vi "WriteFile.vi"(6 "Refresh Time":dbl, 8 "Error In":errorcluster, 9 "Measurements":T1 {"Measurement Type (0: Voltage RMS L-N)" items=["Voltage RMS L-N", "Voltage RMS L-L", "Frequency", "Current RMS", "Current Peak", "Crest Factor", "Power Factor", "Power VA", "Real Power", "Voltage Harmonic THD", "Voltage Harmonic OHD", "Voltage Harmonic EHD", "Current Harmonic THD", "Current Harmonic OHD", "Current Harmonic EHD"]; "Channel Name(1: A)" items=["A"=1, "B"=2, "C"=3]}, 10 "Load Settings":T2 {"Arbitrary Waveform"."Waveform Number (2: Arbitrary Waveform2)" items=["Arbitrary Waveform 2"=2, "Arbitrary Waveform 3"=3, "Arbitrary Waveform 4"=4, "Arbitrary Waveform 5"=5, "Arbitrary Waveform 6"=6, "Arbitrary Waveform 7"=7, "Arbitrary Waveform 8"=8, "Arbitrary Waveform 9"=9, "Arbitrary Waveform 10"=10, "Arbitrary Waveform 11"=11, "Arbitrary Waveform 12"=12, "Arbitrary Waveform 13"=13, "Arbitrary Waveform 14"=14, "Arbitrary Waveform 15"=15, "Arbitrary Waveform 16"=16, "Arbitrary Waveform 17"=17, "Arbitrary Waveform 18"=18, "Arbitrary Waveform 19"=19, "Arbitrary Waveform 20"=20, "Arbitrary Waveform 21"=21, "Arbitrary Waveform 22"=22]; "Waveform"."Waveform (1: Sine)" items=["Sine"=1, "Arbitrary Waveform 2"=2, "Arbitrary Waveform 3"=3, "Arbitrary Waveform 4"=4, "Arbitrary Waveform 5"=5, "Arbitrary Waveform 6"=6, "Arbitrary Waveform 7"=7, "Arbitrary Waveform 8"=8, "Arbitrary Waveform 9"=9, "Arbitrary Waveform 10"=10, "Arbitrary Waveform 11"=11, "Arbitrary Waveform 12"=12, "Arbitrary Waveform 13"=13, "Arbitrary Waveform 14"=14, "Arbitrary Waveform 15"=15, "Arbitrary Waveform 16"=16, "Arbitrary Waveform 17"=17, "Arbitrary Waveform 18"=18, "Arbitrary Waveform 19"=19, "Arbitrary Waveform 20"=20, "Arbitrary Waveform 21"=21, "Arbitrary Waveform 22"=22]; "Waveform"."Channel Name (1: A)" items=["A"=1, "B"=2, "C"=3]; "Frequency"."Frequency Range (600Hz)" items=["150 Hz", "300 Hz", "600 Hz", "1200 Hz"]; "Range Control (0: Auto)" items=["Auto", "<110 V", "110 V -120.9 V", "121 V - 130.9 V", "> 131 V"]; "Configure Output"."Form (3: Three)" items=["Single", "Split", "Three"]; "Configure Output"."Coupling  (0: Direct)" items=["Direct", "Transformer"]}, 11 "refnum":T3) -> (0 "error out":errorcluster)   [LabVIEW 2018, in "AcPwrPlugins.lvlib" / "PacificPowerSource.lvclass"]
doc: "This VI writes the properties to the INI configuration file."
uses:
  PacificPowerSource.lvclass
  <vilib>/Utility/config.llb/Config Data RefNum.ctl
  TypeDefs/DeviceSettings.ctl
  TypeDefs/Measurements.ctl
  <vilib>/Utility/config.llb/NI_LVConfig.lvlib
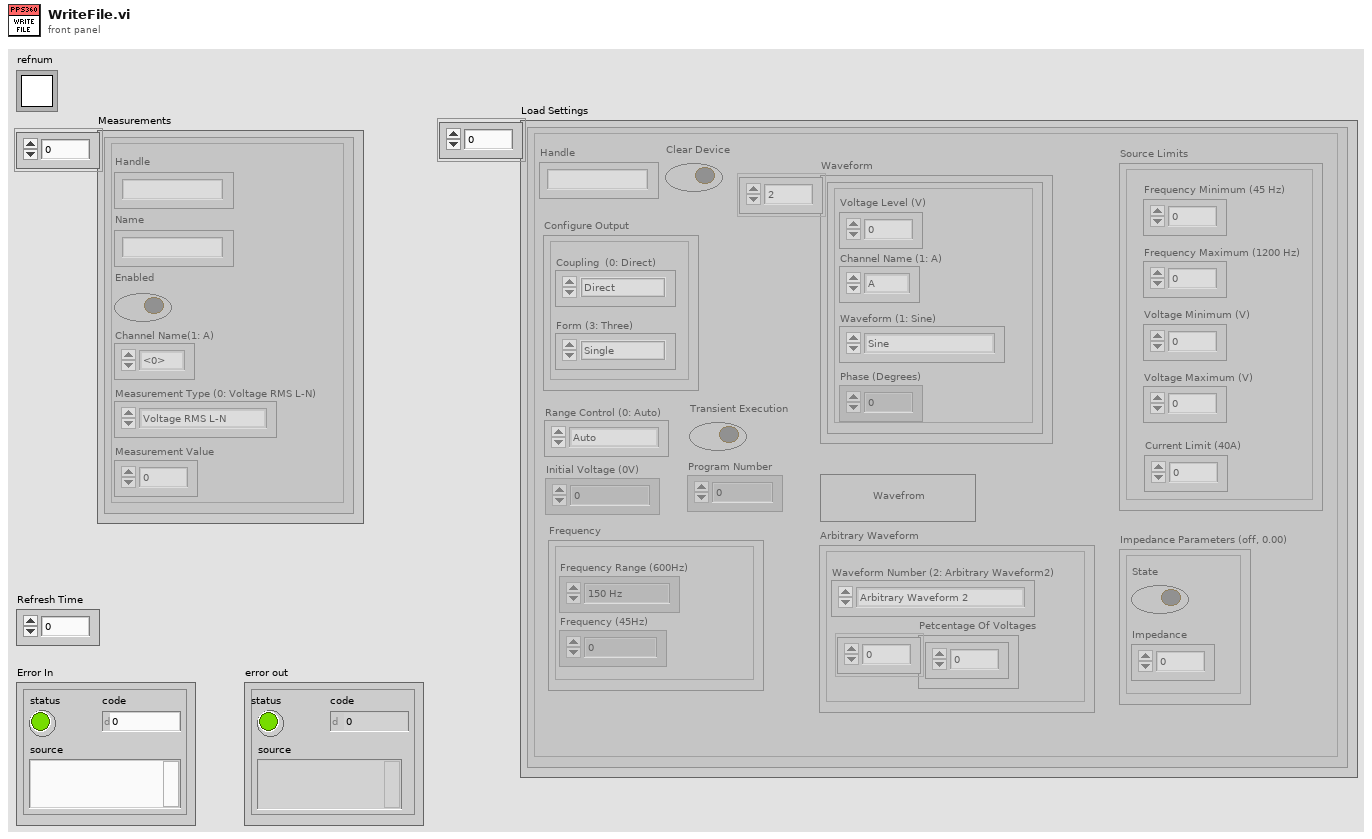
[diagram p1: front panel]
types:
  T1 = typedef "AcPwrPlugins.lvlib/PacificPowerSource.lvclass/Measurements.ctl" = cluster{"Handle":string, "Name":string, "Enabled":bool, "Measurement Value":dbl, "Channel Name(1: A)":u16, "Measurement Type (0: Voltage RMS L-N)":u16}[]
  T2 = typedef "AcPwrPlugins.lvlib/PacificPowerSource.lvclass/DeviceSettings.ctl" = cluster{"Handle":string, "Connected":bool, "Source Limits":cluster{"Frequency Minimum (45 Hz)":dbl, "Frequency Maximum (1200 Hz)":dbl, "Voltage Maximum (V)":dbl, "Voltage Minimum (V)":dbl, "Current Limit (40A)":dbl}, "Clear Device":bool, "Configure Output":cluster{"Coupling  (0: Direct)":u16, "Form (3: Three)":u16}, "Range Control (0: Auto)":u16, "Initial Voltage (0V)":u16, "Frequency":cluster{"Frequency Range (600Hz)":u16, "Frequency (45Hz)":dbl}, "Waveform":cluster{"Voltage Level (V)":dbl, "Phase (Degrees)":i32, "Channel Name (1: A)":u16, "Waveform (1: Sine)":u16}[], "Arbitrary Waveform":cluster{"Waveform Number (2: Arbitrary Waveform2)":u16, "Petcentage Of Voltages":dbl[]}, "Impedance Parameters (off, 0.00)":cluster{"State":bool, "Impedance":dbl}, "Waveform Type":bool, "Program Number":i32, "Transient Execution":bool}[]
  T3 = typedef "NI_LVConfig.lvlib/Config Data RefNum.ctl" = refnum<k1>
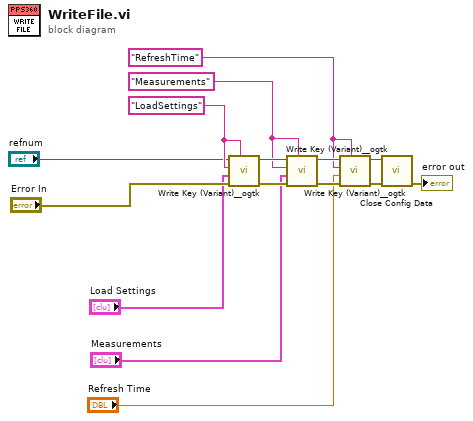
[diagram p0: block diagram]
diagram:
  w7 = "Measurements" ("section (optional)")
  w10 = "RefreshTime" ("section (optional)")
  w11 = "LoadSettings" ("section (optional)")
  n1 = call <userlib>:"Write Key (Variant)__ogtk.vi"("section"=w11, "error in (no error)"="Error In", "key-value"="Load Settings", "key (optional)"=w11, "refnum"="refnum") -> ("error out"=w14:errorcluster, "refnum out"=w15:T3)  [unwired: 5 in]
  n2 = call <userlib>:"Write Key (Variant)__ogtk.vi"("section"=w7, "error in (no error)"=w14, "key-value"="Measurements", "key (optional)"=w7, "refnum"=w15) -> ("error out"=w12:errorcluster, "refnum out"=w13:T3)  [unwired: 5 in]
  n3 = call <userlib>:"Write Key (Variant)__ogtk.vi"("section"=w10, "error in (no error)"=w12, "key-value"="Refresh Time", "key (optional)"=w10, "refnum"=w13) -> ("error out"=w8:errorcluster, "refnum out"=w9:T3)  [unwired: 5 in]
  n4 = call <vilib>:"Close Config Data.vi"("error in (no error)"=w8, "refnum"=w9) -> ("error out"=→"error out":errorcluster)  [unwired: 8 in, 1 out]
